vi "Initialization VI.vi"(8 "error in (no error)":errorcluster, 10 "Custom XML":string, 11 "Device Item Ref in":T1 format="%.0x") -> (0 "error out":errorcluster, 3 "Device Item Ref out":T1 format="%.0x")   [LabVIEW 2019, in "WaveFormCustomDevice System Explorer.lvlib"]
uses:
  WaveFormCustomDevice System Explorer.lvlib
  <vilib>/NI VeriStand/Custom Device API/Custom Device Item Ref.ctl
  <vilib>/NI VeriStand/Custom Device API/Custom Device Channel.ctl
  <vilib>/NI VeriStand/Custom Device API/Custom Device Channel Type.ctl
  <vilib>/NI VeriStand/Custom Device API/Custom Device API.lvlib
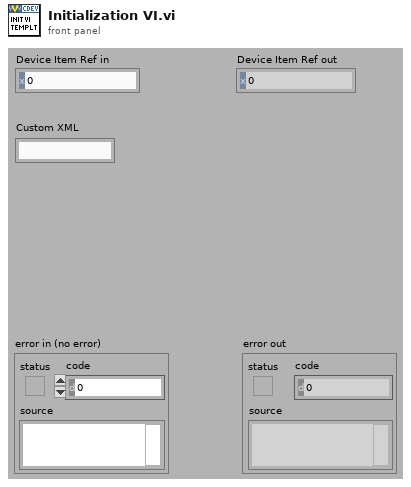
[diagram p1: front panel]
types:
  T1 = typedef "Custom Device API.lvlib/Custom Device Item Ref.ctl" = u64
  T2 = typedef "Custom Device API.lvlib/Custom Device Channel.ctl" = cluster{"Type":T3, "Units":string, "Default Value":dbl, "Faultable":bool, "Scalable":bool}
  T3 = typedef "Custom Device API.lvlib/Custom Device Channel Type.ctl" = enum16{"Input", "Output"}
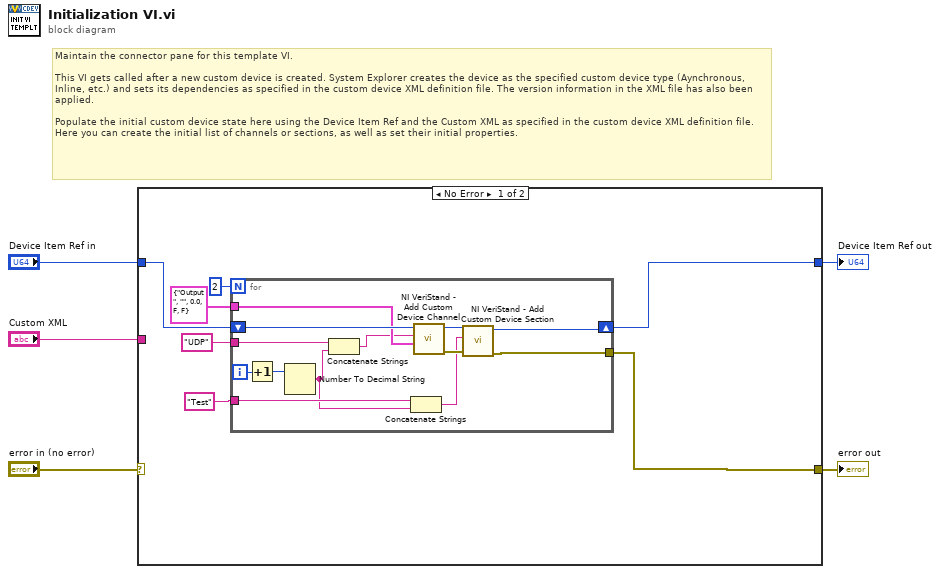
[diagram p0: block diagram]
diagram:
  # "Maintain the connector pane for this template VI.\n\nThis VI gets called after a new custom device is created. System Explorer creates the device as the specified custom device type (Aynchronous, Inline, etc.) and sets its dependencies as specified in the custom device XML definition file. The version information in the XML file has also been applied.\n\nPopulate the initial custom device state here using the Device Item Ref and the Custom XML as specified in the custom device XML definition file. Here you can create the initial list of channels or sections, as well as set their initial properties."
  n1 = case shown="No Error" "error in (no error)" {
    selector: "error in (no error)" -> [_ w27]
    tunnel: [w6 w27] -> w5
    tunnel: [w8 w26] -> w3
    tunnel: "Device Item Ref in" -> [w12 w26]
    tunnel: "Custom XML" -> [_ _]
    frame No Error {
      n2 = for {
        N: 2 -> [_]
        tunnel: T2 {"Type"=enum."Output", "Units"="", "Default Value"=0.0, "Faultable"=FALSE, "Scalable"=FALSE} ("Channel") -> [w24]
        shift-right: [w14] -> w8
        shift-left: w12 -> [w25]
        tunnel: "UDP" ("Channel Name") -> [w21]
        tunnel: "Test" ("Section Name") -> [w16]
        tunnel: [w13] -> w6
        i -> [w20]
        n3 = Increment(x=w20) -> (x+1=w19:i32)
        n4 = Number To Decimal String(number=w19) -> (decimal integer string=w15:string)  [unwired: 1 in]
        n5 = Concatenate Strings(w21, w15) -> (w18:string)
        n6 = Concatenate Strings(w16, w15) -> (w17:string)
        n7 = call <vilib>:"NI VeriStand - Add Custom Device Channel.vi"("Channel"=w24, "Channel Name"=w18, "Parent Ref in"=w25) -> ("error out"=w23:errorcluster, "Parent Ref out"=w22:T1)  [unwired: 5 in, 2 out]
        n8 = call <vilib>:"NI VeriStand - Add Custom Device Section.vi"("error in (no error)"=w23, "Section Name"=w17, "Parent Ref in"=w22) -> ("error out"=w13:errorcluster, "Parent Ref out"=w14:T1)  [unwired: 5 in, 2 out]
      }
    }
    frame Error {
    }
  }
  "error out" <- w5
  "Device Item Ref out" <- w3
